vi "Change Setpoint.vi"(8 "error in (no error)":errorcluster, 10 "Setpoint":dbl, 11 "Alicat Device in":refnum<class "Alicat Device.lvclass">) -> (0 "error out":errorcluster, 3 "Alicat Device out":refnum<class "Alicat Device.lvclass">)   [LabVIEW 2015, in "Alicat Lib.lvlib" / "Alicat Device.lvclass"]
uses:
  Alicat Device.lvclass
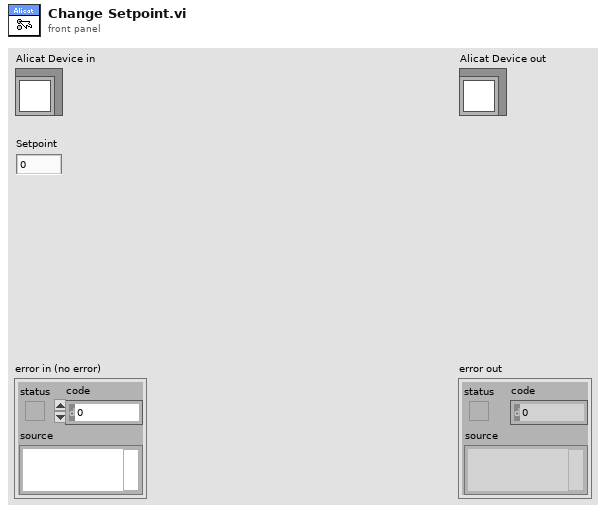
[diagram p1: front panel]
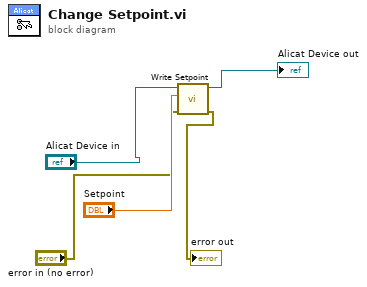
[diagram p0: block diagram]
diagram:
  n1 = call "Write Setpoint.vi"("error in"="error in (no error)", "Setpoint"="Setpoint", "Alicat Device in"="Alicat Device in") -> ("error out"=→"error out":errorcluster, "Alicat Device out"=→"Alicat Device out":refnum<class "Alicat Device.lvclass">)  [unwired: 6 in, 1 out]
